vi "Init Front Panel.vi"(8 "error in":errorcluster, 11 "VI Reference":refnum<vi>) -> (0 "error out":errorcluster)   [LabVIEW 2021]
doc: "Initialises or sets up the user-facing front panel (GUI) of the application.\nIncludes:\n1. Setting up the area of the front panel that is displayed to the user\n2. Opening or displaying the front panel"
uses:
  <vilib>/Utility/miscctls.llb/LVPointTypeDef.ctl
  <vilib>/Utility/miscctls.llb/LVRectTypeDef.ctl
panel:
  # "Development\ncontrols/indicators useful for development and testing, but which are not outputs of the VI"
  # "Input\nInputs to the VI"
  # "Output\nOutputs of the VI"
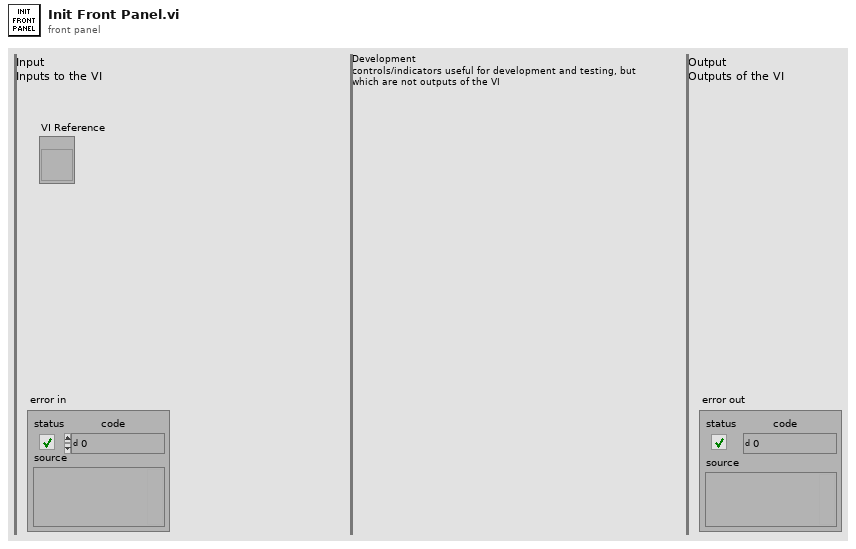
[diagram p1: front panel]
types:
  T1 = enum32{"Invalid", "Standard", "Closed", "Hidden", "Minimized", "Maximized"}
  T2 = typedef "LVRectTypeDef.ctl" = cluster{"Left":i16, "Top":i16, "Right":i16, "Bottom":i16}
  T3 = typedef "LVPointTypeDef.ctl" = cluster{"Horizontal":i16, "Vertical":i16}
  T4 = enum16{"Always On", "Always Off", "Off While Running"}
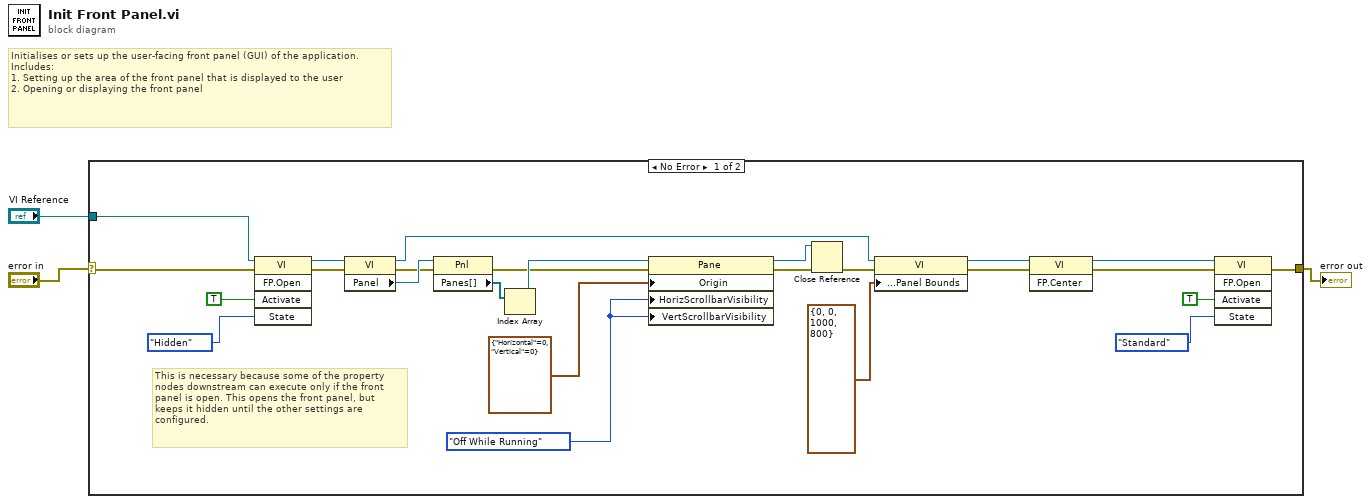
[diagram p0: block diagram]
diagram:
  # "Initialises or sets up the user-facing front panel (GUI) of the application.\nIncludes:\n1. Setting up the area of the front panel that is displayed to the user\n2. Opening or displaying the front panel"
  n1 = case shown="No Error" "error in" {
    selector: "error in" -> [w12 w29]
    tunnel: [w15 w29] -> w2
    tunnel: "VI Reference" -> [w11 _]
    frame No Error {
      w4 = T4."Off While Running" ("Horizontal Scrollbar Visibility")
      # "This is necessary because some of the property nodes downstream can execute only if the front panel is open. This opens the front panel, but keeps it hidden until the other settings are configured."
      n2 = invoke class="VI" method="FP.Open"(reference=w11, error in=w12, "Activate"=TRUE ("Activate?"), "State"=T1."Hidden") -> (reference out=w9:refnum<vi>, error out=w10:errorcluster)  [unwired: 1 in, 3 out]
      n3 = property class="VI"(reference=w9, error in=w10) -> (reference out=w19:refnum<vi>, error out=w23:errorcluster, "Panel"=w26:refnum<vi>)
      n4 = property class="Pnl"(reference=w26, error in=w23) -> (error out=w22:errorcluster, "Panes[]"=w25:refnum<vi>[])  [unwired: 1 out]
      n5 = Index Array(array=w25) -> (element=w24:refnum<vi>)  [unwired: 1 in]
      n6 = property class="Pane"(reference=w24, error in=w22, "Origin"=T3 {"Horizontal"=0, "Vertical"=0}, "HorizScrollbarVisibility"=w4, "VertScrollbarVisibility"=w4) -> (reference out=w17:refnum<vi>, error out=w20:errorcluster)
      n7 = Close Reference(reference=w17, error in (no error)=w20) -> (error out=w18:errorcluster)
      n8 = property on="Property Node" class="VI"(reference=w19, error in=w18, "Front Panel Window:Panel Bounds"=T2 {"Left"=0, "Top"=0, "Right"=1000, "Bottom"=800}) -> (reference out=w8:refnum<vi>, error out=w6:errorcluster)
      n9 = invoke class="VI" method="FP.Center"(reference=w8, error in=w6) -> (reference out=w7:refnum<vi>, error out=w5:errorcluster)  [unwired: 1 in, 1 out]
      n10 = invoke class="VI" method="FP.Open"(reference=w7, error in=w5, "Activate"=TRUE ("Activate?"), "State"=T1."Standard") -> (error out=w15:errorcluster)  [unwired: 1 in, 4 out]
    }
    frame Error {
    }
  }
  "error out" <- w2
